vi "Get AQS.vi"(0 "NMR in":refnum<class "NMR.lvclass">, 11 "error in (no error)":errorcluster) -> (4 "NMR out":refnum<class "NMR.lvclass">, 6 "Real Data":i32[](array[numeric]), 8 "Imag Data":i32[](array[numeric]), 15 "error out":errorcluster)   [LabVIEW 2011, in "NMR.lvclass"]
uses:
  NMR.lvclass
panel:
  out "String as ASCII":string
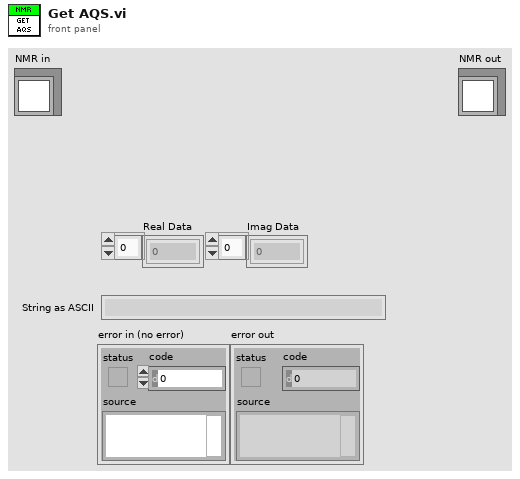
[diagram p1: front panel]
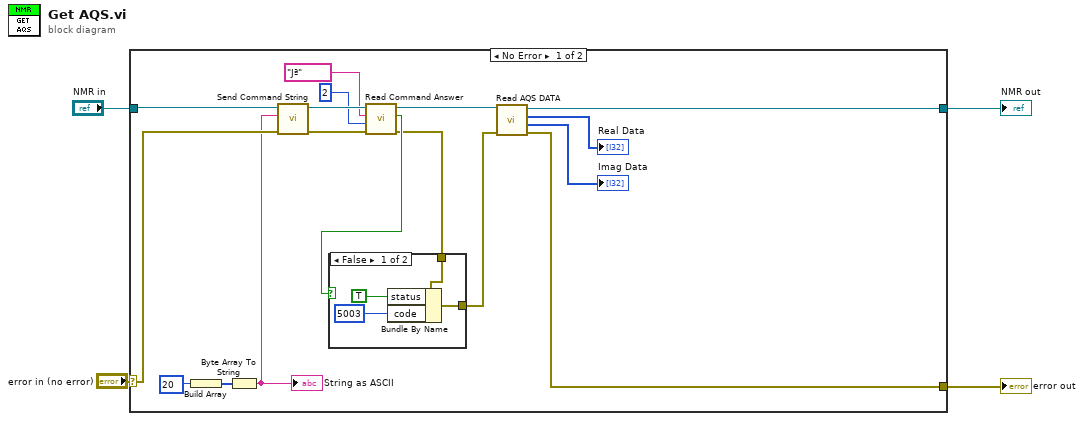
[diagram p0: block diagram]
diagram:
  n1 = case shown="No Error" "error in (no error)" {
    selector: "error in (no error)" -> [w20 w28]
    tunnel: [w7 w28] -> w3
    tunnel: [w11 w27] -> w1
    tunnel: "NMR in" -> [w10 w27]
    frame No Error {
      n2 = Build Array(u32 20 ("element")) -> (w18:u32[])
      n3 = Byte Array To String(unsigned byte array=w18) -> (string=w16:string)
      "String as ASCII" <- w16
      n4 = call-dynamic "Send Command String.vi"("error in (no error)"=w20, "Command String"=w16, "NMR in"=w10) -> ("error out"=w19:errorcluster, "NMR out"=w21:refnum<class "NMR.lvclass">)  [unwired: 7 in]
      n5 = call-dynamic "Read Command Answer.vi"("error in (no error)"=w19, "bytes to read"=u32 2 ("Number bytes Read"), "String Seached"="Jª" ("search char"), "NMR in"=w21) -> ("error out"=w12:errorcluster, "Expected Answer?"=w13:bool, "NMR out"=w9:refnum<class "NMR.lvclass">)  [unwired: 5 in]
      n6 = case shown="False" w13 {
        tunnel: w12 -> [w23 w26]
        tunnel: [w22 w26] -> w8
        frame False {
          n7 = Bundle By Name(cluster=w23, "status"=TRUE, "code"=5003) -> (w22:errorcluster)
        }
        frame True {
        }
      }
      n8 = call-dynamic "Read AQS DATA.vi"("error in (no error)"=w8, "NMR in"=w9) -> ("error out"=w7:errorcluster, "Imag Data"=→"Imag Data":i32[], "Real Data"=→"Real Data":i32[], "NMR out"=w11:refnum<class "NMR.lvclass">)  [unwired: 5 in, 1 out]
    }
    frame Error {
    }
  }
  "error out" <- w3
  "NMR out" <- w1
